vi "create temp folders.vi"(8 "error in (no error)":errorcluster, 11 "a3Di stations":enum16{"APG", "Inspection", "Diagnostic"}[](array[ring])) -> (0 "error out":errorcluster, 3 "Temporary folders":path[](array[path]))   [LabVIEW 2013, in "Manipulate IPF.lvlib"]
uses:
  Manipulate IPF.lvlib
  <vilib>/Utility/sysdir.llb/System Directory Type.ctl
  <userlib>/_OpenG.lib/file/file.llb/File Exists - Scalar__ogtk.vi
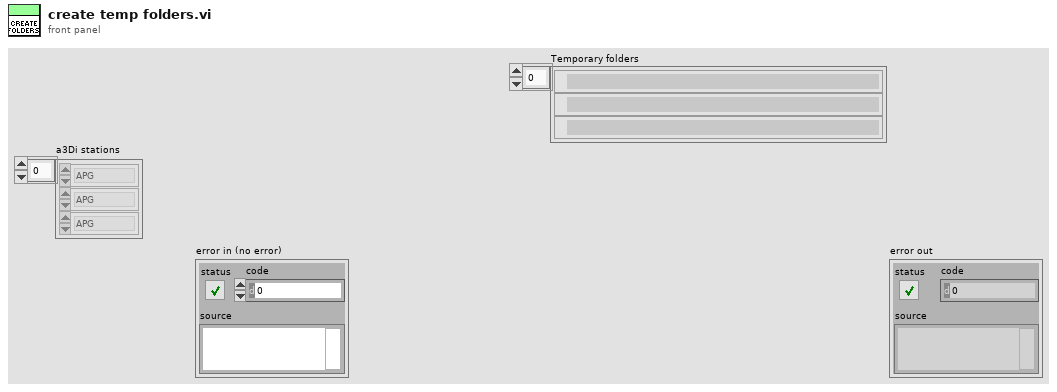
[diagram p1: front panel]
types:
  T1 = typedef "System Directory Type.ctl" = i32
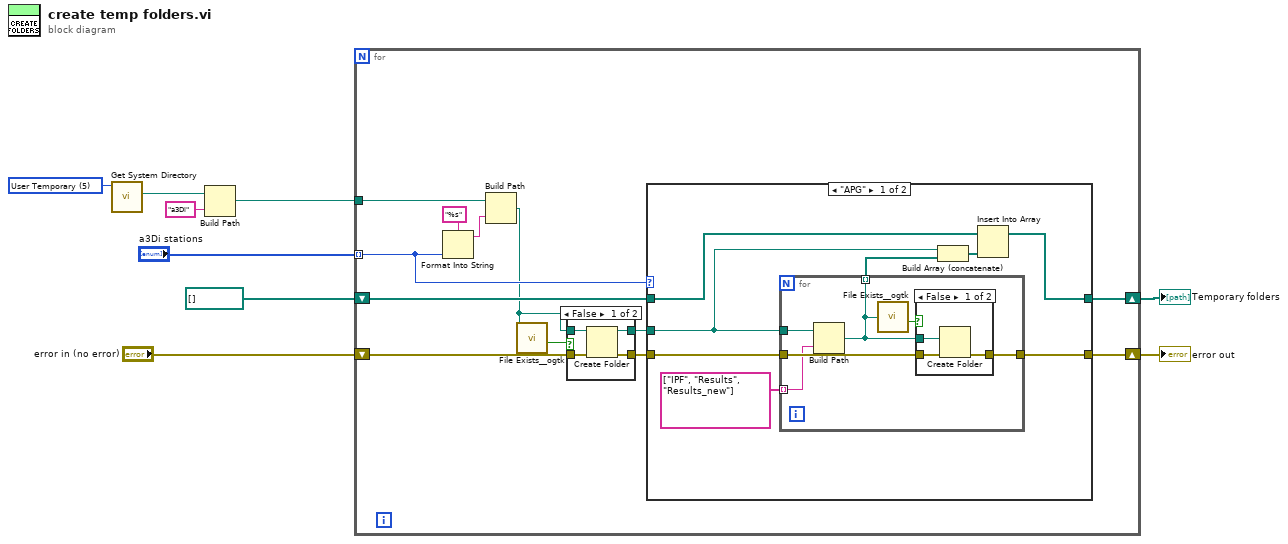
[diagram p0: block diagram]
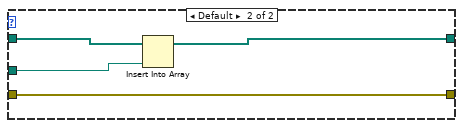
[diagram p4: hidden frame]
diagram:
  w9 = T1 5 items=["User Home"=0, "User Desktop"=1, "User Documents"=2, "User Application Data"=3, "User Preferences"=4, "User Temporary"=5, "Public Documents"=6, "Public Application Data"=7, "Public Preferences"=8, "Public Cache"=13, "System Core Libraries"=9, "System Installed Libraries"=10, "Application Files"=11, "Boot Volume Root"=12] ("system directory type")
  n1 = call <vilib>:"Get System Directory.vi"("system directory type"=w9) -> ("system directory"=w6:path)  [unwired: 10 in]
  n2 = Build Path(base path=w6, name or relative path="a3Di") -> (appended path=w5:path)
  n3 = for {
    shift-right: [w16] -> w8
    shift-left: "error in (no error)" -> [w21]
    tunnel: w5 -> [w20]
    tunnel: "a3Di stations" -> [w15] mode=indexing
    shift-right: [w13] -> w1
    shift-left: path[] [] -> [w14]
    n4 = Format Into String(format string="%s", w15) -> (resulting string=w19:string)  [unwired: 2 in, 1 out]
    n5 = Build Path(base path=w20, name or relative path=w19) -> (appended path=w10:path)
    n6 = call-poly <userlib>:"File Exists__ogtk.vi"("file path"=w10) -> ("exists"=w12:bool)  [unwired: 6 in, 1 out]
    n7 = case shown="False" w12 {
      tunnel: w10 -> [w25 w27]
      tunnel: w21 -> [w24 w26]
      tunnel: [w22 w26] -> w17
      tunnel: [w23 w27] -> w11
      frame False {
        n8 = Create Folder(path (use dialog)=w25, error in=w24) -> (created path=w23:path, error out=w22:errorcluster)  [unwired: 1 in, 1 out]
      }
      frame True {
      }
    }
    n9 = case shown="\"APG\"" w15 {
      tunnel: w11 -> [w31 w48]
      tunnel: w17 -> [w35 w49]
      tunnel: [w30 w49] -> w16
      tunnel: w14 -> [w32 w47]
      tunnel: [w33 w46] -> w13
      frame "APG" {
        n10 = for {
          tunnel: w35 -> [w41]
          tunnel: w31 -> [w40]
          tunnel: [w39] -> w30
          tunnel: [w38] -> w29 mode=indexing
          tunnel: string[] ["IPF", "Results", "Results_new"] -> [w36] mode=indexing
          n11 = Build Path(base path=w40, name or relative path=w36) -> (appended path=w38:path)
          n12 = call-poly <userlib>:"File Exists__ogtk.vi"("file path"=w38) -> ("exists"=w37:bool)  [unwired: 6 in, 1 out]
          n13 = case shown="False" w37 {
            tunnel: w41 -> [w44 w45]
            tunnel: [w43 w45] -> w39
            tunnel: w38 -> [w42 _]
            frame False {
              n14 = Create Folder(path (use dialog)=w42, error in=w44) -> (error out=w43:errorcluster)  [unwired: 1 in, 2 out]
            }
            frame True {
            }
          }
        }
        n15 = Build Array (concatenate)(w31, w29) -> (w34:path[])
        n16 = Insert Into Array(array=w32, new element=w34) -> (w33:path[])  [unwired: 1 in]
      }
      frame Default {
        n17 = Insert Into Array(array=w47, new element=w48) -> (w46:path[])  [unwired: 1 in]
      }
    }
  }
  "error out" <- w8
  "Temporary folders" <- w1
